vi "Aero_Tunnel_Monitor.vi"() -> ()   [LabVIEW 2012]
uses:
  ATE_Road_Data.ctl
  ATE_Machine_Status.ctl
  ATE_Road_Control.ctl
  ATE_Balance_Data.ctl
  ATE_Fan_Control.ctl
  ATE_Fan_Data.ctl
  Controls/Post_Process.ctl
  <vilib>/Platform/TimedLoop/XDataNode/timing_clust.ctl
  <vilib>/Platform/TimedLoop/XDataNode/nitl_modes.ctl
  <vilib>/Platform/TimedLoop/XDataNode/wakeup.ctl
  ADAM Client/Sub VIs/ADAM Controls/Update_scan_value.ctl
  Globals/Meas_global.vi
  <vilib>/Platform/TimedLoop/XDataNode/XDataNode.xnode
  <vilib>/Platform/TimedLoop/XDataNode/XDNodeRunTimeDep.lvlib
panel:
  out "Dem Tunnel Speed":dbl
  out "Paths":path[](array[path])
  out "error out":errorcluster
  out "Road Data REF":refnum<k21>="ni.var.psp://192.168.8.2/ATE_Shared_Variables/Road_Data"
  out "Road Control REF":refnum<k21>="ni.var.psp://192.168.8.2/ATE_Shared_Variables/Road_Control"
  out "Fan Data REF":refnum<k21>="ni.var.psp://192.168.8.2/ATE_Shared_Variables/Fan_Data"
  out "Fan Control REF":refnum<k21>="ni.var.psp://192.168.8.2/ATE_Shared_Variables/Fan_Control"
  out "Balance Data REF":refnum<k21>="ni.var.psp://192.168.8.2/ATE_Shared_Variables/Balance_Data"
  out "ATE_Machine Status REF":refnum<k21>="ni.var.psp://192.168.8.2/ATE_Shared_Variables/ATE_Machine_Status"
  in  "Stop Button":bool
  out "SMAD Temp":dbl=22.85
  out "First Loop? 3":bool
  out "First Loop? 2":bool
  out "First Loop?":bool=TRUE
  out "Fan Data":T1={"Fan Speed Dial (RPM)"=1.0, "Wind Speed Dial (m/s)"=0.0, "Wind Speed (m/s)"=0.0, "Fan Speed (RPM)"=1.0} {"Wind Speed Dial (m/s)" scale=0.0..45.0; "Fan Speed Dial (RPM)" scale=0.0..1000.0}
  out "Fan Control":T2={"Reset Pitot?"=FALSE, "Set Fan State"=FALSE, "Set Pressure"=1006.6041, "Set Fan Speed"=0.0, "Set Wind Speed Ratio"=0.0, "Tweak Change?"=FALSE, "Speed Change?"=FALSE}
  out "Balance_Data":T3={"%Lift"=28.01, "Lift"=185.018, "%Pitch"=22.34, "Pitch"=18.53, "%Drag"=2.21, "Drag"=4.327, "%Side"=-0.01, "Side"=-0.05, "%Yaw"=-2.47, "Yaw"=-0.307, "%Roll"=0.55, "Roll"=0.455} {"%Roll" scale=-100.0..100.0; "Roll" format="%5.1f Nm"; "%Yaw" scale=-100.0..100.0; "Yaw" format="%5.1f Nm"; "%Side" scale=-100.0..100.0; "Side" format="%5.1f N"; "%Drag" scale=-100.0..100.0; "Drag" format="%5.1f N"; "%Pitch" scale=-100.0..100.0; "Pitch" format="%5.1f Nm"; "%Lift" scale=-100.0..100.0; "Lift" format="%5.1f N"}
  in  "Road Control":T4 {"BL Suction Fan 2" scale=0.0..100.0; "BL Suction Fan 1" scale=0.0..100.0}
  out "ATE_Machine_Status":T5={"Loop Status"=FALSE, "Loop Frequency"=321.8613369862449, "Poor Loops"=0.0, "Pulse"=TRUE} {"Poor Loops" format="%0.2f %"; "Loop Frequency" format="%0.2f Hz"}
  out "Motor Enable":bool=TRUE
  out "Fan Watchdog":bool
  in  "Display Graph?":bool
  out "Belt Slip Warning":bool
  out "Road Enabled":bool
  out "Working Section Temperature":dbl=23.0
  out "Dem Road Speed":dbl
  in  "Balance Safety Limits":T6(array[cluster])=[{"Max +ve Range"=80, "Min -ve Range"=80, "Axis"="Lift"}, {"Max +ve Range"=80, "Min -ve Range"=80, "Axis"="Pitch"}, {"Max +ve Range"=120, "Min -ve Range"=120, "Axis"="Drag"}, {"Max +ve Range"=80, "Min -ve Range"=80, "Axis"="Side"}, {"Max +ve Range"=120, "Min -ve Range"=120, "Axis"="Yaw"}, {"Max +ve Range"=80, "Min -ve Range"=80, "Axis"="Roll"}]
  in  "Menu Ring":u16(ring) items=["Lift", "Pitch", "Drag", "Side", "Yaw", "Roll"]
  out "Waveform Chart":dbl(graph)
  out "OGI Client Loop Status":T5={"Loop Status"=FALSE, "Loop Frequency"=341.33991618739697, "Poor Loops"=1.2012012012012012, "Pulse"=FALSE} {"Poor Loops" format="%0.2f %"; "Loop Frequency" format="%0.2f Hz"}
  out "Road_Data":T7 {"Road Speed" scale=0.0..50.0; "Yaw Angle" scale=-5.0..5.0}
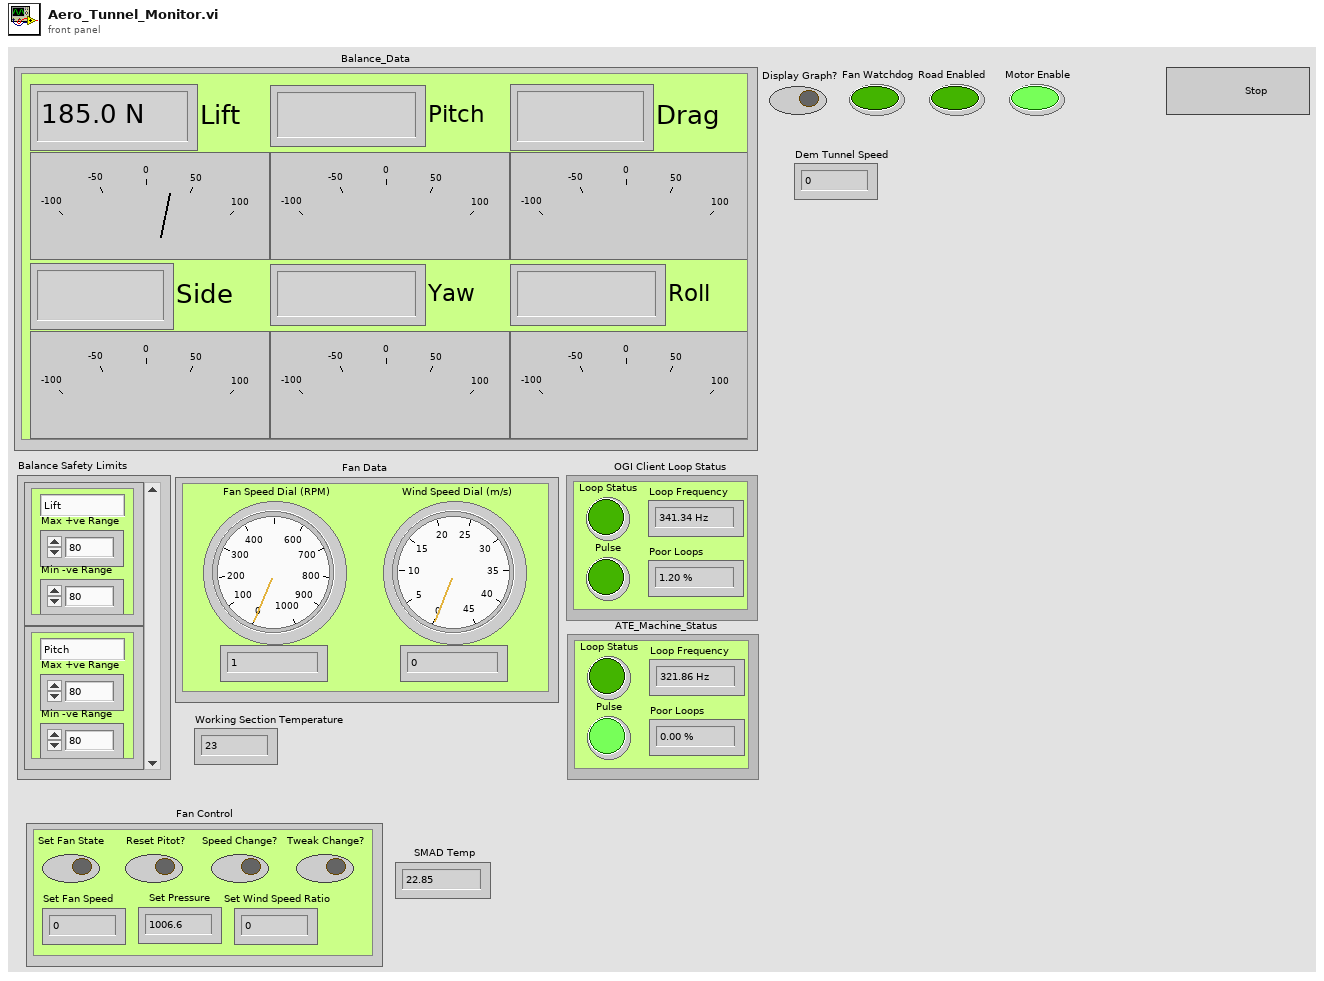
[diagram p1: front panel]
types:
  T1 = cluster{"Fan Speed Dial (RPM)":dbl, "Wind Speed Dial (m/s)":dbl, "Wind Speed (m/s)":dbl, "Fan Speed (RPM)":dbl}
  T2 = typedef "ATE_Fan_Control.ctl" = cluster{"Reset Pitot?":bool, "Set Fan State":bool, "Set Pressure":dbl, "Set Fan Speed":dbl, "Set Wind Speed Ratio":dbl, "Tweak Change?":bool, "Speed Change?":bool}
  T3 = typedef "ATE_Balance_Data.ctl" = cluster{"%Lift":dbl, "Lift":dbl, "%Pitch":dbl, "Pitch":dbl, "%Drag":dbl, "Drag":dbl, "%Side":dbl, "Side":dbl, "%Yaw":dbl, "Yaw":dbl, "%Roll":dbl, "Roll":dbl}
  T4 = typedef "ATE_Road_Control.ctl" = cluster{"Sync to Wind":bool, "Start Drive":bool, "Stop Drive":bool, "BL Suction Fan 1":i32, "BL Suction Fan 2":i32, "Set Yaw Angle":dbl, "Road Active?":bool}
  T5 = typedef "ATE_Machine_Status.ctl" = cluster{"Loop Status":bool, "Loop Frequency":dbl, "Poor Loops":dbl, "Pulse":bool}
  T6 = cluster{"Max +ve Range":i32, "Min -ve Range":i32, "Axis":string}[]
  T7 = typedef "ATE_Road_Data.ctl" = cluster{"Road Information":string, "Road Status":string, "Yaw Angle":dbl, "Road Speed":dbl}
  T8 = typedef "Post_Process.ctl" = enum16{"Take New Data", "Post Process Raw Data File"}
  T9 = typedef "Update_scan_value.ctl" = cluster{"Channel Name":string, "New Value":dbl}
  T10 = typedef "XDNodeRunTimeDep.lvlib/timing_clust.ctl" = cluster{"Expected End [f-1]":u64, "Actual End [f-1]":u64, "Finished Late? [f-1]":bool, "Expected End [i-1]":u64, "Actual End [i-1]":u64, "Finished Late? [i-1]":bool, "Expected Start [i]":u64, "Actual Start [i]":u64, "Expected Start [f]":u64, "Actual Start [f]":u64, "Source Name":string, "Structure Name":string, "Period":i64, "Deadline":i64, "Offset":i64, "Start":i64, "Priority":i32, "Timeout":i32, "Mode":T11, "Wakeup Reason":T12, "Error":errorcluster, "Source Type":string, "Secondary Source Type":string, "Global End Time":u64, "Global Start Time":u64, "Frame Duration":u64, "Iteration Duration":u64, "Assigned CPU":i32, "I/O Scan Engine Mode":u32}
  T11 = typedef "XDNodeRunTimeDep.lvlib/nitl_modes.ctl" = enum32{"No Change", "Process missed periods, maintain original phase", "Discard missed periods, maintain original phase", "Process missed periods, ignore original phase", "Discard missed periods, ignore original phase"}
  T12 = typedef "XDNodeRunTimeDep.lvlib/wakeup.ctl" = enum32{"Normal", "Aborted", "Asynchronous wakeup", "Timing source error", "Timed loop error", "Timeout"}
  T13 = typedef "ATE_Fan_Data.ctl" = cluster{"Fan Speed (RPM)":dbl, "Wind Speed (m/s)":dbl, "SMAD Data":string}
  T14 = typedef "LVDateTimeRec.ctl" = cluster{"fractional second":dbl, "second":i32, "minute":i32, "hour":i32, "day of month":i32, "month":i32, "year":i32, "day of week":i32, "day of year":i32, "DST":i32}
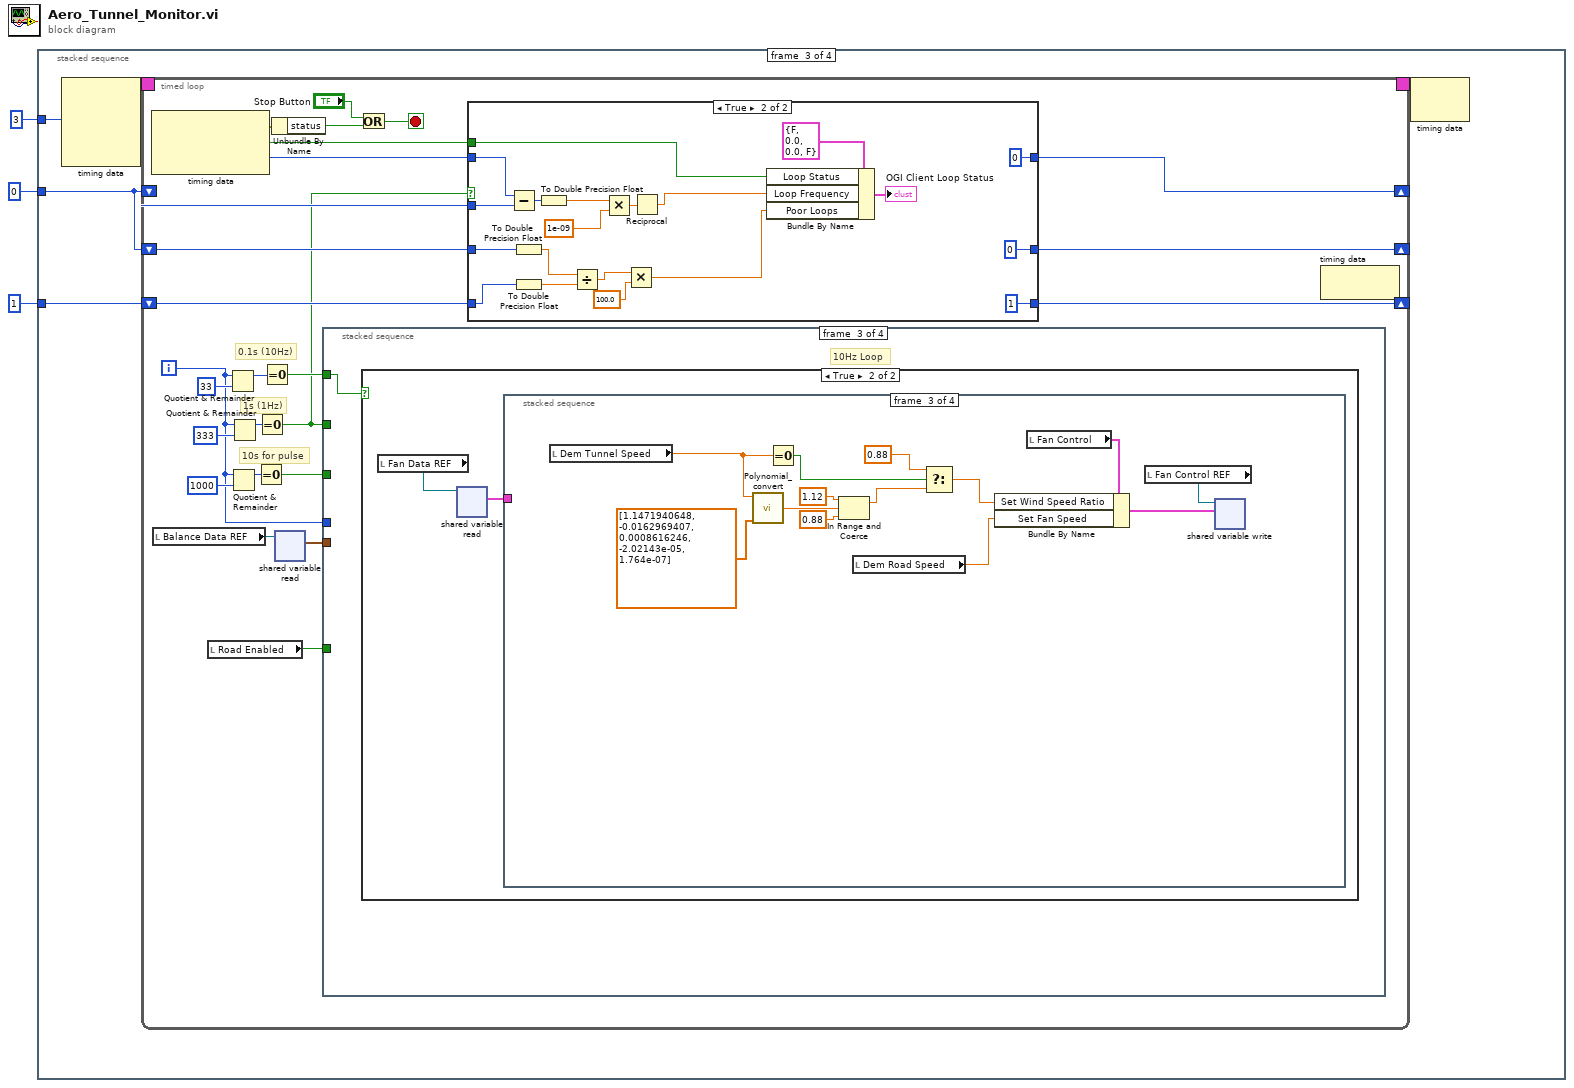
[diagram p0: block diagram]
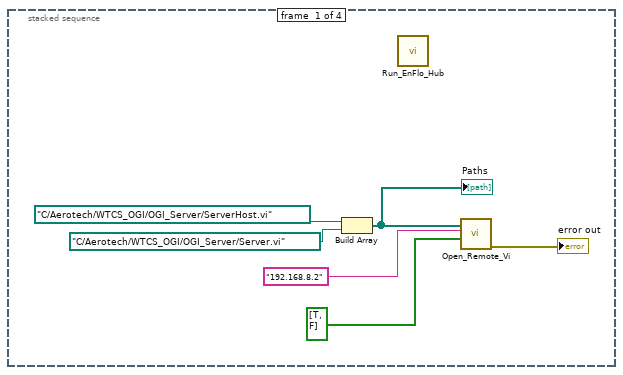
[diagram p2: hidden frame]
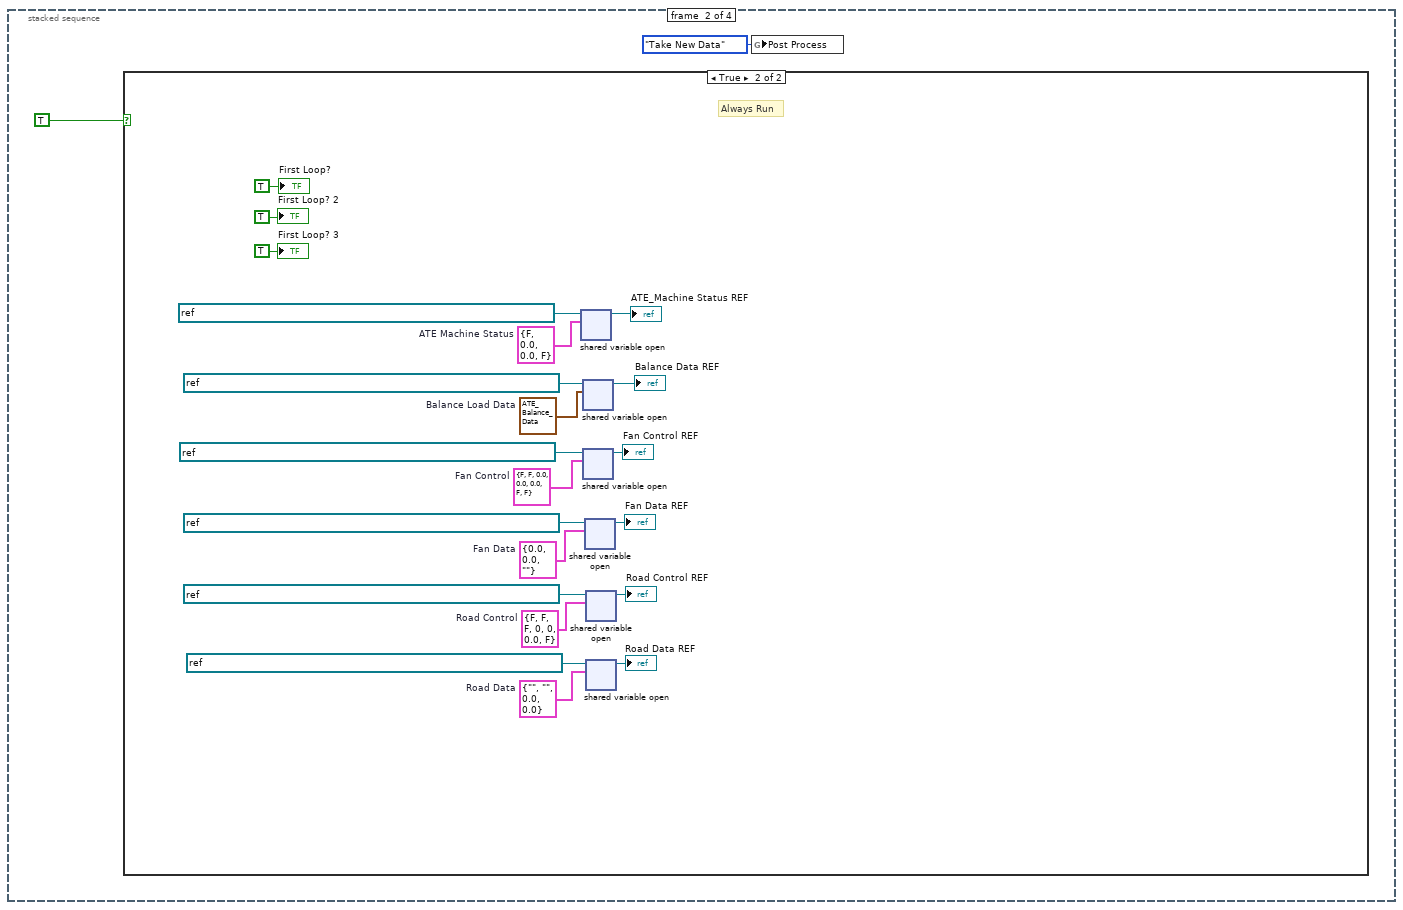
[diagram p3: hidden frame]
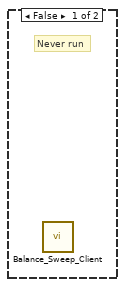
[diagram p4: hidden frame]
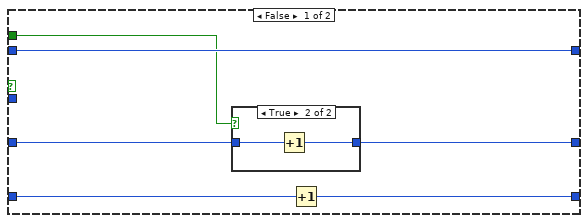
[diagram p5: hidden frame]
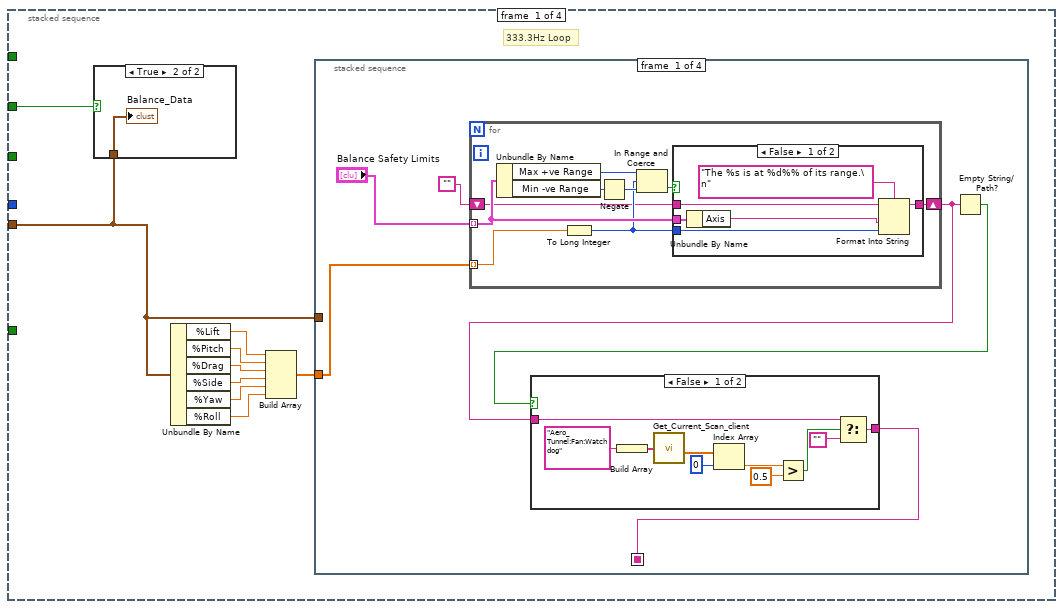
[diagram p7: hidden frame]
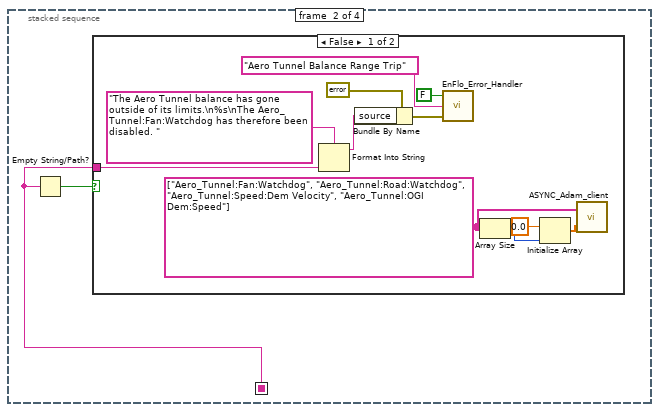
[diagram p11: hidden frame]
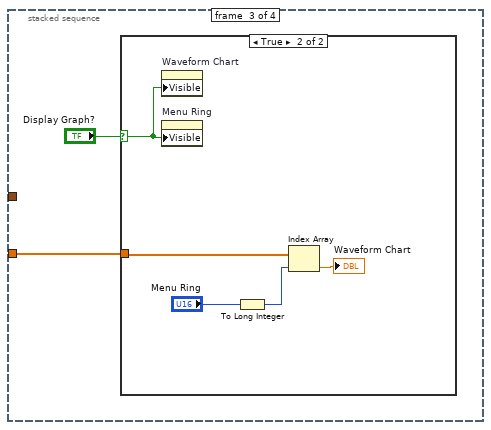
[diagram p13: hidden frame]
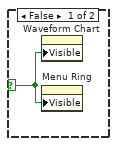
[diagram p14: hidden frame]
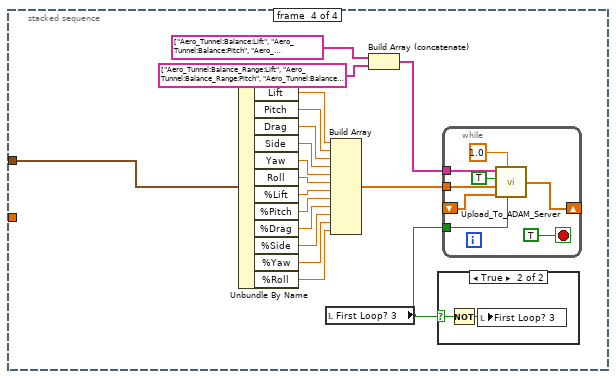
[diagram p15: hidden frame]
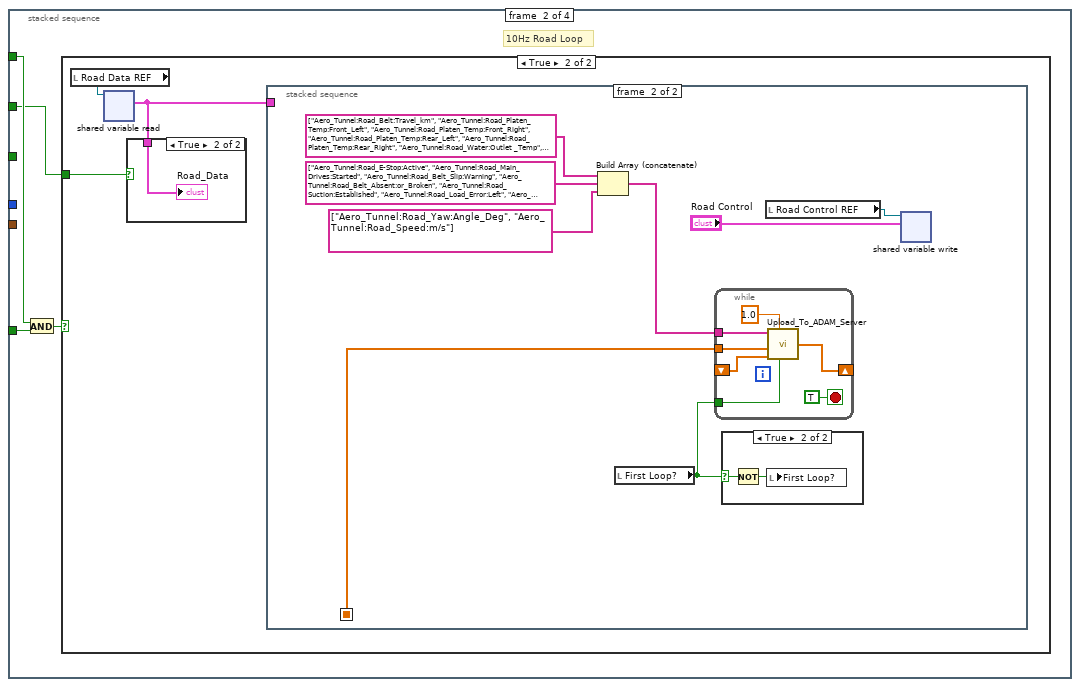
[diagram p17: hidden frame]
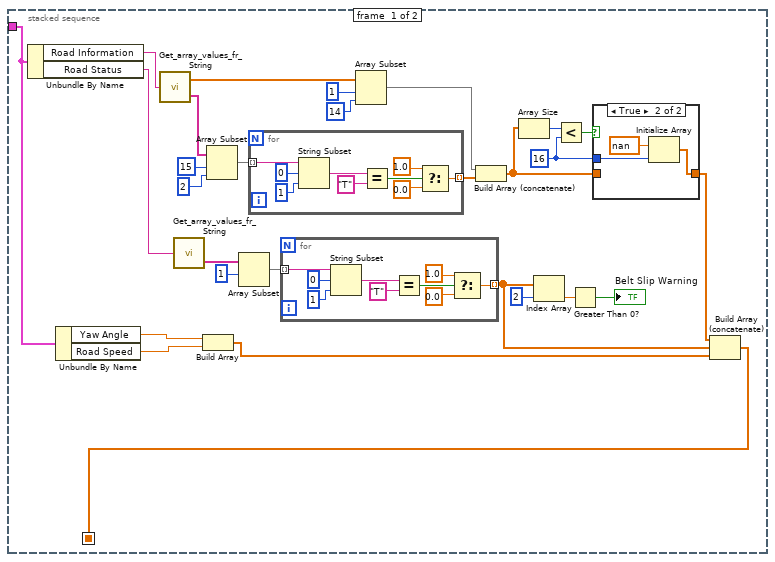
[diagram p20: hidden frame]
diagram:
  n1 = stacked-sequence {
    tunnel: i64 3 ("Period") -> [_ _ w35 _]
    tunnel: i64 0 ("Period") -> [_ _ w34 _]
    tunnel: i64 1 ("Period") -> [_ _ w33 _]
    frame #0 {
      n2 = Build Array(path "C:/Aerotech/WTCS_OGI/OGI_Server/ServerHost.vi" ("VI Path"), path "C:/Aerotech/WTCS_OGI/OGI_Server/Server.vi" ("VI Path")) -> (w6:path[])
      "Paths" <- w6
      n3 = call "Run_EnFlo_Hub.vi"() -> ()  [unwired: 8 in]
      n4 = call "Open_Remote_Vi.vi"("Run Minimised?"=bool[] [TRUE, FALSE], "Remote IP"="192.168.8.2", "Vi Path"=w6) -> ("error out"=→"error out":errorcluster)  [unwired: 8 in]
    }
    frame #1 {
      n5 = case shown="True" TRUE {
        frame False {
          # "Never run"
          n6 = call "Balance_Sweep_Client.vi"() -> ()  [unwired: 5 in, 1 out]
        }
        frame True {
          w16 = T7 {"Road Information"="", "Road Status"="", "Yaw Angle"=0.0, "Road Speed"=0.0}  # Road Data
          w18 = T4 {"Sync to Wind"=FALSE, "Start Drive"=FALSE, "Stop Drive"=FALSE, "BL Suction Fan 1"=0, "BL Suction Fan 2"=0, "Set Yaw Angle"=0.0, "Road Active?"=FALSE}  # Road Control
          w28 = T5 {"Loop Status"=FALSE, "Loop Frequency"=0.0, "Poor Loops"=0.0, "Pulse"=FALSE}  # ATE Machine Status
          w20 = T13 {"Fan Speed (RPM)"=0.0, "Wind Speed (m/s)"=0.0, "SMAD Data"=""}  # Fan Data
          w22 = T2 {"Reset Pitot?"=FALSE, "Set Fan State"=FALSE, "Set Pressure"=0.0, "Set Fan Speed"=0.0, "Set Wind Speed Ratio"=0.0, "Tweak Change?"=FALSE, "Speed Change?"=FALSE}  # Fan Control
          w26 = T3 {"%Lift"=0.0, "Lift"=0.0, "%Pitch"=0.0, "Pitch"=0.0, "%Drag"=0.0, "Drag"=0.0, "%Side"=0.0, "Side"=0.0, "%Yaw"=0.0, "Yaw"=0.0, "%Roll"=0.0, "Roll"=0.0}  # Balance Load Data
          # "Always Run"
          n7 = shared-variable-open(refnum<k21> "ni.var.psp://192.168.8.2/ATE_Shared_Variables/ATE_Machine_Status" ("shared variable refnum in"), w28) -> (→"ATE_Machine Status REF":refnum<k21>)  [unwired: 2 in, 1 out]
          n8 = shared-variable-open(refnum<k21> "ni.var.psp://192.168.8.2/ATE_Shared_Variables/Balance_Data" ("shared variable refnum in"), w26) -> (→"Balance Data REF":refnum<k21>)  [unwired: 2 in, 1 out]
          n9 = shared-variable-open(refnum<k21> "ni.var.psp://192.168.8.2/ATE_Shared_Variables/Fan_Control" ("shared variable refnum in"), w22) -> (→"Fan Control REF":refnum<k21>)  [unwired: 2 in, 1 out]
          n10 = shared-variable-open(refnum<k21> "ni.var.psp://192.168.8.2/ATE_Shared_Variables/Fan_Data" ("shared variable refnum in"), w20) -> (→"Fan Data REF":refnum<k21>)  [unwired: 2 in, 1 out]
          n11 = shared-variable-open(refnum<k21> "ni.var.psp://192.168.8.2/ATE_Shared_Variables/Road_Control" ("shared variable refnum in"), w18) -> (→"Road Control REF":refnum<k21>)  [unwired: 2 in, 1 out]
          n12 = shared-variable-open(refnum<k21> "ni.var.psp://192.168.8.2/ATE_Shared_Variables/Road_Data" ("shared variable refnum in"), w16) -> (→"Road Data REF":refnum<k21>)  [unwired: 2 in, 1 out]
          "First Loop?" <- TRUE
          "First Loop? 2" <- TRUE
          "First Loop? 3" <- TRUE
        }
      }
      n13 = global write "Meas_global.vi" "Post Process"(Post_Process."Take New Data" ("Post Process")) -> ()
    }
    frame #2 {
      n14 = node-c288(w35) -> (w37:T10)  [unwired: 3 in]
      n15 = timed-loop {
        timing: w37 -> [_]
        timing-out: [_] -> w36
        shift-right: [w44] -> _
        shift-left: w34 -> [w51]
        shift-right: [w46] -> _
        shift-left: w34 -> [w58]
        shift-right: [w49] -> _
        shift-left: w33 -> [w48]
        i -> [w38]
        stop <- w41 stop-if-true
        # "10s for pulse"
        # "1s (1Hz)"
        # "0.1s (10Hz)"
        n16 = node-c288() -> (w62:errorcluster, w47:bool, w59:i64)  [unwired: 1 in]
        n17 = local read "Balance Data REF"() -> (w40:refnum<k21>)
        n18 = local read "Road Enabled"() -> (w55:bool)
        n19 = Quotient & Remainder(x=w38, y=33) -> (x-y*floor(x/y)=w60:i32)  [unwired: 1 out]
        n20 = Quotient & Remainder(x=w38, y=1000) -> (x-y*floor(x/y)=w56:i32)  [unwired: 1 out]
        n21 = Quotient & Remainder(x=w38, y=333) -> (x-y*floor(x/y)=w61:i32)  [unwired: 1 out]
        n22 = Equal To 0?(x=w56) -> (x = 0?=w50:bool)
        n23 = Equal To 0?(x=w61) -> (x = 0?=w45:bool)
        n24 = Equal To 0?(x=w60) -> (x = 0?=w57:bool)
        n25 = Unbundle By Name(w62) -> ("status"=w43:bool)
        n26 = shared-variable-read(w40) -> (w39:T3)  [unwired: 1 in, 3 out]
        n27 = stacked-sequence {
          tunnel: w57 -> [_ w185 w259 _]
          tunnel: w45 -> [w93 w184 _ _]
          tunnel: w55 -> [_ w186 _ _]
          tunnel: w50 -> [_ _ _ w360]
          tunnel: w39 -> [w92 _ _ _]
          tunnel: w38 -> [_ _ _ w359]
          frame #0 {
            # "333.3Hz Loop"
            n28 = case shown="True" w93 {
              tunnel: w92 -> [_ w101]
              frame False {
              }
              frame True {
                "Balance_Data" <- w101
              }
            }
            n29 = Unbundle By Name(w92) -> ("%Lift"=w99:dbl, "%Pitch"=w98:dbl, "%Drag"=w97:dbl, "%Side"=w96:dbl, "%Yaw"=w95:dbl, "%Roll"=w94:dbl)
            n30 = Build Array(w99, w98, w97, w96, w95, w94) -> (w100:dbl[])
            n31 = stacked-sequence {
              seq-local: [w102 _ _ _] -> [_ w135 _ _]
              tunnel: w100 -> [w106 _ w148 _]
              tunnel: w92 -> [_ _ _ w159]
              frame #0 {
                n32 = for {
                  tunnel: "Balance Safety Limits" -> [w122] mode=indexing
                  tunnel: w106 -> [w125] mode=indexing
                  shift-right: [w119] -> w104
                  shift-left: "" -> [w120]
                  n33 = Unbundle By Name(w122) -> ("Max +ve Range"=w127:i32, "Min -ve Range"=w126:i32)
                  n34 = To Long Integer(number=w125) -> (32bit integer=w121:i32)
                  n35 = Negate(x=w126) -> (-x=w124:i32)
                  n36 = In Range and Coerce(upper limit=w127, x=w121, lower limit=w124) -> (In Range?=w123:bool)  [unwired: 1 out]
                  n37 = case shown="False" w123 {
                    tunnel: w122 -> [w133 _]
                    tunnel: w121 -> [w131 _]
                    tunnel: w120 -> [w129 w134]
                    tunnel: [w128 w134] -> w119
                    frame False {
                      n38 = Unbundle By Name(w133) -> ("Axis"=w132:string)
                      n39 = Format Into String(format string="The %s is at %d%% of its range.\n", initial string=w129, w132, w131) -> (resulting string=w128:string)  [unwired: 1 in, 1 out]
                    }
                    frame True {
                    }
                  }
                }
                n40 = Empty String/Path?(string/path=w104) -> (empty?=w105:bool)
                n41 = case shown="False" w105 {
                  tunnel: w104 -> [w110 w118]
                  tunnel: [w108 w118] -> w102
                  frame False {
                    n42 = Build Array("Aero_Tunnel:Fan:Watchdog") -> (w117:string[])
                    n43 = call "Get_Current_Scan_client.vi"("ADAM Ch Names"=w117) -> ("Numerical Values"=w115:dbl[])  [unwired: 1 in, 2 out]
                    n44 = Index Array(array=w115, index=0) -> (element=w113:dbl)
                    n45 = Greater?(x=w113, y=0.5) -> (0:w111:bool)
                    n46 = Select(t=w110, s=w111, f="") -> (s? t:f=w108:string)
                  }
                  frame True {
                  }
                }
              }
              frame #1 {
                n47 = Empty String/Path?(string/path=w135) -> (empty?=w136:bool)
                n48 = case shown="False" w136 {
                  tunnel: w135 -> [w141 _]
                  frame False {
                    w140 = string[] ["Aero_Tunnel:Fan:Watchdog", "Aero_Tunnel:Road:Watchdog", "Aero_Tunnel:Speed:Dem Velocity", "Aero_Tunnel:OGI Dem:Speed"] ("Channel Names")
                    n49 = Format Into String(format string="The Aero Tunnel balance has gone outside of its limits.\n%s\nThe Aero_Tunnel:Fan:Watchdog has therefore been disabled. ", w141) -> (resulting string=w142:string)  [unwired: 2 in, 1 out]
                    n50 = Bundle By Name(cluster=errorcluster {"status"=TRUE, "code"=0, "source"=""} ("error in (no error)"), "source"=w142) -> (w144:errorcluster)
                    n51 = call "EnFlo_Error_Handler.vi"("error in (no error)"=w144, "Error Type"="Aero Tunnel Balance Range Trip", "Dialog Box (T)"=FALSE) -> ()  [unwired: 3 out]
                    n52 = Array Size(array=w140) -> (size(s)=w139:i32)
                    n53 = Initialize Array(0.0, w139) -> (w137:dbl[])
                    n54 = call "ASYNC_Adam_client.vi"("Values"=w137, "Channel Names"=w140) -> ()  [unwired: 2 out]
                  }
                  frame True {
                  }
                }
              }
              frame #2 {
                n55 = case shown="True" "Display Graph?" {
                  selector: "Display Graph?" -> [w150 w153]
                  tunnel: w148 -> [_ w151]
                  frame False {
                    n56 = property on="Waveform Chart" class="WFChart (strict)"("Visible"=w150) -> ()  [unwired: 2 in, 2 out]
                    n57 = property on="Menu Ring" class="Ring (strict)"("Visible"=w150) -> ()  [unwired: 2 in, 2 out]
                  }
                  frame True {
                    n58 = property on="Waveform Chart" class="WFChart (strict)"("Visible"=w153) -> ()  [unwired: 2 in, 2 out]
                    n59 = property on="Menu Ring" class="Ring (strict)"("Visible"=w153) -> ()  [unwired: 2 in, 2 out]
                    n60 = To Long Integer(number="Menu Ring") -> (32bit integer=w152:i32)
                    n61 = Index Array(array=w151, index=w152) -> (element=→"Waveform Chart":dbl)
                  }
                }
              }
              frame #3 {
                n62 = Unbundle By Name(w159) -> ("Lift"=w173:dbl, "Pitch"=w172:dbl, "Drag"=w171:dbl, "Side"=w170:dbl, "Yaw"=w169:dbl, "Roll"=w168:dbl, "%Lift"=w167:dbl, "%Pitch"=w166:dbl, "%Drag"=w165:dbl, "%Side"=w164:dbl, "%Yaw"=w163:dbl, "%Roll"=w162:dbl)
                n63 = local read "First Loop? 3"() -> (w156:bool)
                n64 = Build Array(w173, w172, w171, w170, w169, w168, w167, w166, w165, w164, w163, w162) -> (w157:dbl[])
                n65 = Build Array (concatenate)(string[] ["Aero_Tunnel:Balance:Lift", "Aero_Tunnel:Balance:Pitch", "Aero_Tunnel:Balance:Drag", "Aero_Tunnel:Balance:Side-Force", "Aero_Tunnel:Balance:Yaw", "Aero_Tunnel:Balance:Roll"] ("Channel Names"), string[] ["Aero_Tunnel:Balance_Range:Lift", "Aero_Tunnel:Balance_Range:Pitch", "Aero_Tunnel:Balance_Range:Drag", "Aero_Tunnel:Balance_Range:Side-Force", "Aero_Tunnel:Balance_Range:Yaw", "Aero_Tunnel:Balance_Range:Roll"] ("Channel Names")) -> (w158:string[])
                n66 = case shown="True" w156 {
                  selector: w156 -> [_ w175]
                  frame False {
                  }
                  frame True {
                    n67 = Not(x=w175) -> (.not. x?=w174:bool)
                    n68 = local write "First Loop? 3"(w174) -> ()
                  }
                }
                n69 = while {
                  tunnel: w158 -> [w183]
                  tunnel: w157 -> [w181]
                  shift-right: [w179] -> _
                  shift-left: _ -> [w178]
                  tunnel: w156 -> [w177]
                  stop <- TRUE stop-if-true
                  n70 = call "Upload_To_ADAM_Server.vi"("First Loop"=w177, "Averaging Period (s)"=1.0, "Shift In"=w178, "Channel Values"=w181, "Give Variance"=TRUE, "Channel Names"=w183) -> ("Shift Out"=w179:dbl[])
                }
              }
            }
          }
          frame #1 {
            # "10Hz Road Loop"
            n71 = And(x=w185, y=w186) -> (x .and. y?=w187:bool)
            n72 = case shown="True" w187 {
              tunnel: w184 -> [_ w190]
              frame False {
                # "Do Nothing"
              }
              frame True {
                n73 = local read "Road Data REF"() -> (w189:refnum<k21>)
                n74 = shared-variable-read(w189) -> (w188:T7)  [unwired: 1 in, 3 out]
                n75 = case shown="True" w190 {
                  tunnel: w188 -> [_ w191]
                  frame False {
                  }
                  frame True {
                    "Road_Data" <- w191
                  }
                }
                n76 = stacked-sequence {
                  seq-local: [w196 _] -> [_ w245]
                  tunnel: w188 -> [w195 _]
                  frame #0 {
                    w217 = 16 ("y")
                    n77 = Unbundle By Name(w195) -> ("Road Information"=w206:string, "Road Status"=w200:string)
                    n78 = Unbundle By Name(w195) -> ("Yaw Angle"=w194:dbl, "Road Speed"=w193:dbl)
                    n79 = call "Get_array_values_fr_String.vi"("String Value"=w206) -> ("Numeric Array"=w218:dbl[], "String array"=w214:string[])
                    n80 = call "Get_array_values_fr_String.vi"("String Value"=w200) -> ("String array"=w203:string[])  [unwired: 1 out]
                    n81 = Build Array(w194, w193) -> (w192:dbl[])
                    n82 = Array Subset(array=w214, index=15, length=2) -> (w211:string[])
                    n83 = Array Subset(array=w203, index=1) -> (w205:string[])  [unwired: 1 in]
                    n84 = for {
                      tunnel: w211 -> [w239] mode=indexing
                      tunnel: [w233] -> w212 mode=indexing
                      n85 = String Subset(string=w239, offset (0)=0, length (rest)=1 ("length (rest)")) -> (substring=w238:string)
                      n86 = Equal?(x=w238, y="T") -> (x = y?=w236:bool)
                      n87 = Select(t=1.0, s=w236, f=0.0) -> (s? t:f=w233:dbl)
                    }
                    n88 = for {
                      tunnel: [w221] -> w197 mode=indexing
                      tunnel: w205 -> [w220] mode=indexing
                      n89 = String Subset(string=w220, offset (0)=0, length (rest)=1 ("length (rest)")) -> (substring=w226:string)
                      n90 = Equal?(x=w226, y="T") -> (x = y?=w224:bool)
                      n91 = Select(t=1.0, s=w224, f=0.0) -> (s? t:f=w221:dbl)
                    }
                    n92 = Array Subset(array=w218, index=1, length=14) -> (w213:dbl[])
                    n93 = Build Array (concatenate)(w213, w212) -> (w219:dbl[])
                    n94 = Array Size(array=w219) -> (size(s)=w215:i32)
                    n95 = Index Array(array=w197, index=2) -> (element=w202:dbl)
                    n96 = Less?(x=w215, y=w217) -> (x < y?=w216:bool)
                    n97 = Greater Than 0?(x=w202) -> (x > 0?=→"Belt Slip Warning":bool)
                    n98 = case shown="True" w216 {
                      tunnel: [w229 w232] -> w198
                      tunnel: w219 -> [w229 _]
                      tunnel: w217 -> [_ w230]
                      frame False {
                      }
                      frame True {
                        n99 = Initialize Array(nan, w230) -> (w232:dbl[])
                      }
                    }
                    n100 = Build Array (concatenate)(w198, w197, w192) -> (w196:dbl[])
                  }
                  frame #1 {
                    n101 = Build Array (concatenate)(string[] ["Aero_Tunnel:Road_Belt:Travel_km", "Aero_Tunnel:Road_Platen_Temp:Front_Left", "Aero_Tunnel:Road_Platen_Temp:Front_Right", "Aero_Tunnel:Road_Platen_Temp:Rear_Left", "Aero_Tunnel:Road_Platen_Temp:Rear_Right", "Aero_Tunnel:Road_Water:Outlet _Temp", "Aero_Tunnel:Road_Water:Inlet _Temp", "Aero_Tunnel:Road_Suction:Front", "Aero_Tunnel:Road_Suction:Middle", "Aero_Tunnel:Road_Suction:Rear", "Aero_Tunnel:Road_BL_Suction:Primary", "Aero_Tunnel:Road_BL_Suction:Secondary", "Aero_Tunnel:Road_LoadCell:Left", "Aero_Tunnel:Road_LoadCell:Right", "Aero_Tunnel:Road_Water_High:Temp_Alarm", "Aero_Tunnel:Road_Platen_High:Temp_Alarm"] ("Channel Names"), string[] ["Aero_Tunnel:Road_E-Stop:Active", "Aero_Tunnel:Road_Main_Drives:Started", "Aero_Tunnel:Road_Belt_Slip:Warning", "Aero_Tunnel:Road_Belt_Absent:or_Broken", "Aero_Tunnel:Road_Suction:Established", "Aero_Tunnel:Road_Load_Error:Left", "Aero_Tunnel:Road_Load_Error:Right", "Aero_Tunnel:Road_Water_Alarm:Active", "Aero_Tunnel:Road_Platen_Alarm:Active"] ("Channel Names"), string[] ["Aero_Tunnel:Road_Yaw:Angle_Deg", "Aero_Tunnel:Road_Speed:m/s"] ("Channel Names")) -> (w246:string[])
                    n102 = local read "First Loop?"() -> (w244:bool)
                    n103 = while {
                      tunnel: w246 -> [w258]
                      tunnel: w245 -> [w256]
                      shift-right: [w254] -> _
                      shift-left: _ -> [w253]
                      tunnel: w244 -> [w252]
                      stop <- TRUE stop-if-true
                      n104 = call "Upload_To_ADAM_Server.vi"("First Loop"=w252, "Averaging Period (s)"=1.0, "Shift In"=w253, "Channel Values"=w256, "Channel Names"=w258) -> ("Shift Out"=w254:dbl[])  [unwired: 1 in]
                    }
                    n105 = case shown="True" w244 {
                      selector: w244 -> [_ w251]
                      frame False {
                      }
                      frame True {
                        n106 = Not(x=w251) -> (.not. x?=w250:bool)
                        n107 = local write "First Loop?"(w250) -> ()
                      }
                    }
                    n108 = local read "Road Control REF"() -> (w243:refnum<k21>)
                    n109 = shared-variable-write(w243, "Road Control") -> ()  [unwired: 1 in, 2 out]
                  }
                }
              }
            }
          }
          frame #2 {
            # "10Hz Loop"
            n110 = case shown="True" w259 {
              frame False {
                # "Do Nothing"
              }
              frame True {
                n111 = local read "Fan Data REF"() -> (w261:refnum<k21>)
                n112 = shared-variable-read(w261) -> (w260:T13)  [unwired: 1 in, 3 out]
                n113 = stacked-sequence {
                  tunnel: w260 -> [w284 _ _ _]
                  frame #0 {
                    w270 = 17 ("y")
                    n114 = Unbundle By Name(w284) -> ("Wind Speed (m/s)"=w266:dbl, "Fan Speed (RPM)"=w267:dbl, "SMAD Data"=w268:string)
                    n115 = call "Get_array_values_fr_String.vi"("String Value"=w268) -> ("Numeric Array"=w271:dbl[], "String array"=w274:string[])
                    n116 = Array Size(array=w274) -> (size(s)=w275:i32)
                    n117 = Less?(x=w275, y=w270) -> (x < y?=w273:bool)
                    n118 = case shown="True" w273 {
                      tunnel: [w289 w292] -> w272
                      tunnel: w271 -> [w289 _]
                      tunnel: w270 -> [_ w290]
                      frame False {
                      }
                      frame True {
                        n119 = Initialize Array(nan, w290) -> (w292:dbl[])
                      }
                    }
                    n120 = Bundle By Name(cluster=T1 {"Fan Speed Dial (RPM)"=143.0, "Wind Speed Dial (m/s)"=4.76, "Wind Speed (m/s)"=0.0, "Fan Speed (RPM)"=0.0} ("Fan Data"), "Wind Speed Dial (m/s)"=w266, "Fan Speed Dial (RPM)"=w267, "Wind Speed (m/s)"=w266, "Fan Speed (RPM)"=w267) -> (→"Fan Data":T1)
                    n121 = Index Array(array=w272, index=16) -> (element=w262:dbl)
                    "SMAD Temp" <- w262
                    n122 = Index Array(array=w272, index=1) -> (element=w281:dbl)
                    n123 = Index Array(array=w272, index=11) -> (element=w279:dbl)
                    n124 = Less?(x=w279, y=100.0) -> (x < y?=w277:bool)
                    n125 = Boolean To (0,1)(Boolean=w277) -> (0, 1=w276:i16)
                    n126 = Build Array(w262, w281, w276) -> (w269:dbl[])
                    n127 = local read "First Loop? 2"() -> (w265:bool)
                    n128 = Build Array (concatenate)(w266, w267, w269) -> (w285:dbl[])
                    n129 = case shown="True" w265 {
                      selector: w265 -> [_ w288]
                      frame False {
                      }
                      frame True {
                        n130 = Not(x=w288) -> (.not. x?=w287:bool)
                        n131 = local write "First Loop? 2"(w287) -> ()
                      }
                    }
                    n132 = while {
                      tunnel: string[] ["Aero_Tunnel:Speed:Meas Velocity", "Aero_Tunnel:Fan:RPM", "Aero_Tunnel:SmAD:Temp", "Aero_Tunnel:Pitot tube:Voltage", "Aero_Tunnel:Drive:Ready"] ("Channel Names") -> [w299]
                      tunnel: w285 -> [w297]
                      shift-right: [w296] -> _
                      shift-left: _ -> [w295]
                      tunnel: w265 -> [w293]
                      stop <- TRUE stop-if-true
                      n133 = call "Upload_To_ADAM_Server.vi"("First Loop"=w293, "Averaging Period (s)"=1.0, "Shift In"=w295, "Channel Values"=w297, "Channel Names"=w299) -> ("Shift Out"=w296:dbl[])  [unwired: 1 in]
                    }
                  }
                  frame #1 {
                    n134 = call "Get_Current_Scan_client.vi"("ADAM Ch Names"=string[] ["Aero_Tunnel:Road:Dem_Velocity", "Froude:NPL:Atmos_Press", "Aero_Tunnel:Motor:Enable", "Aero_Tunnel:Thermistor:Temp", "Aero_Tunnel:Fan:Watchdog", "Aero_Tunnel:Rolling_Road:Enable", "Aero_Tunnel:Speed:Dem Velocity"] ("appended array")) -> ("Numerical Values"=w325:dbl[])  [unwired: 1 in, 2 out]
                    n135 = Index Array(array=w325) -> (element #1=w314:dbl, element #2=w318:dbl, element #3=w320:dbl, element #4=→"Working Section Temperature":dbl, element #5=w302:dbl, element #6=w301:dbl, element #7=→"Dem Tunnel Speed":dbl)  [unwired: 7 in]
                    "Dem Road Speed" <- w314
                    n136 = local read "Dem Road Speed"() -> (w317:dbl)
                    n137 = To Unsigned Word Integer(number=w302) -> (unsigned 16bit integer=w323:u16)
                    n138 = To Unsigned Word Integer(number=w301) -> (unsigned 16bit integer=w324:u16)
                    n139 = Greater?(x=w314, y=0.2) -> (0:w313:bool)
                    n140 = Not Equal To 0?(x=w324) -> (x != 0?=w310:bool)
                    "Road Enabled" <- w310
                    n141 = Not Equal To 0?(x=w323) -> (x != 0?=→"Fan Watchdog":bool)
                    n142 = Greater?(x=w320, y=0.5) -> (0:w312:bool)
                    "Motor Enable" <- w312
                    n143 = Not Equal?(x=w314, y=w317) -> (x != y?=w316:bool)
                    n144 = Not(x=w312) -> (.not. x?=w311:bool)
                    n145 = local read "Road Control"() -> (w305:T4)
                    n146 = Bundle By Name(cluster=w305, "Road Active?"=w310) -> (w309:T4)
                    n147 = Bundle By Name(cluster=T2 {"Reset Pitot?"=FALSE, "Set Fan State"=FALSE, "Set Pressure"=0.0, "Set Fan Speed"=0.0, "Set Wind Speed Ratio"=0.0, "Tweak Change?"=FALSE, "Speed Change?"=FALSE} ("Fan Control"), "Set Fan State"=w313, "Speed Change?"=w316, "Set Pressure"=w318, "Reset Pitot?"=w311, "Tweak Change?"=FALSE) -> (w306:T2)
                    "Fan Control" <- w306
                    n148 = local read "Road Control REF"() -> (w308:refnum<k21>)
                    n149 = local read "Fan Control REF"() -> (w307:refnum<k21>)
                    n150 = property on="Road_Data" class="Clust (strict)"("Visible"=w310) -> ()  [unwired: 2 in, 2 out]
                    n151 = property on="Road Control" class="Clust (strict)"("Visible"=w310) -> ()  [unwired: 2 in, 2 out]
                    n152 = property on="Belt Slip Warning" class="Bool (strict)"("Visible"=w310) -> ()  [unwired: 2 in, 2 out]
                    n153 = shared-variable-write(w307, w306) -> ()  [unwired: 1 in, 2 out]
                    n154 = shared-variable-write(w308, w309) -> ()  [unwired: 1 in, 2 out]
                  }
                  frame #2 {
                    n155 = local read "Dem Tunnel Speed"() -> (w332:dbl)
                    n156 = call "Polynomial_convert.vi"("Calib constants"=dbl[] [1.1471940648, -0.0162969407, 0.0008616246, -2.02143e-05, 1.764e-07], "Voltage"=w332) -> ("Eng Values"=w337:dbl)  [unwired: 4 in]
                    n157 = Equal To 0?(x=w332) -> (x = 0?=w331:bool)
                    n158 = In Range and Coerce(upper limit=1.12, x=w337, lower limit=0.88) -> (coerced(x)=w330:dbl)  [unwired: 1 out]
                    n159 = local read "Dem Road Speed"() -> (w327:dbl)
                    n160 = Select(t=0.88, s=w331, f=w330) -> (s? t:f=w329:dbl)
                    n161 = local read "Fan Control"() -> (w335:T2)
                    n162 = Bundle By Name(cluster=w335, "Set Wind Speed Ratio"=w329, "Set Fan Speed"=w327) -> (w334:T2)
                    n163 = local read "Fan Control REF"() -> (w333:refnum<k21>)
                    n164 = shared-variable-write(w333, w334) -> ()  [unwired: 1 in, 2 out]
                  }
                  frame #3 {
                    n165 = while {
                      shift-right: [w341] -> _
                      shift-left: _ -> [w342]
                      stop <- TRUE stop-if-true
                      n166 = local read "Working Section Temperature"() -> (w340:dbl)
                      n167 = Greater?(x=w340, y=35.0) -> (0:w341:bool)
                      n168 = Compound Arithmetic op=AND(invert w342, w341) -> (w347:bool)
                      n169 = Number To Fractional String(number=w340, precision (6)=i16 2) -> (F-format string=w344:string)  [unwired: 2 in]
                      n170 = case shown="True" w347 {
                        tunnel: w344 -> [_ w352]
                        frame False {
                        }
                        frame True {
                          w351 = string[] ["Aero_Tunnel:Fan:Watchdog", "Aero_Tunnel:Road:Watchdog", "Aero_Tunnel:Speed:Dem Velocity", "Aero_Tunnel:OGI Dem:Speed"] ("Channel Names")
                          n171 = Format Into String(format string="The Aero Tunnel temperature has gone above it's limits and is:\n%s\nThe Aero_Tunnel:Fan:Watchdog has therefore been disabled. ", w352) -> (resulting string=w353:string)  [unwired: 2 in, 1 out]
                          n172 = Bundle By Name(cluster=errorcluster {"status"=TRUE, "code"=0, "source"=""} ("error in (no error)"), "source"=w353) -> (w355:errorcluster)
                          n173 = Array Size(array=w351) -> (size(s)=w350:i32)
                          n174 = call "EnFlo_Error_Handler.vi"("error in (no error)"=w355, "Error Type"="Aero Tunnel Temperature Trip", "Dialog Box (T)"=FALSE) -> ()  [unwired: 3 out]
                          n175 = Initialize Array(0.0, w350) -> (w348:dbl[])
                          n176 = call "ASYNC_Adam_client.vi"("Values"=w348, "Channel Names"=w351) -> ()  [unwired: 2 out]
                        }
                      }
                    }
                  }
                }
              }
            }
          }
          frame #3 {
            # "10s Loop For Pulse"
            n177 = case shown="True" w360 {
              tunnel: w359 -> [_ w361]
              frame False {
                # "Do Nothing"
              }
              frame True {
                n178 = while {
                  shift-right: [w366] -> _
                  shift-left: "Start" -> [w367]
                  shift-right: [w365] -> _
                  shift-left: _ -> [w364]
                  tunnel: w361 -> [w363]
                  stop <- w368 continue-if-true
                  n179 = case shown="\"Close Server\"" w367 {
                    tunnel: [FALSE TRUE TRUE TRUE TRUE FALSE] -> w368
                    tunnel: ["" "Check Pulse" "Check Pulse" w408 "ReOpen" ""] -> w366
                    tunnel: [w369 w375 0 ("code") w400 w436 w445] -> w365
                    tunnel: w364 -> [w369 w376 _ w397 w436 w445]
                    tunnel: w363 -> [_ w379 _ _ _ _]
                    frame "No Match", Default {
                    }
                    frame "Start" {
                      n180 = Greater?(x=w379, y=1500) -> (0:w374:bool)
                      n181 = while {
                        shift-right: [w383] -> _
                        shift-left: _ -> [w382]
                        stop <- TRUE stop-if-true
                        n182 = Seconds To Date/Time() -> (date time rec=w384:T14)  [unwired: 2 in]
                        n183 = Unbundle By Name(w384) -> ("day of year"=w383:i32)
                        n184 = Not Equal?(x=w383, y=w382) -> (x != y?=w381:bool)
                        n185 = case shown="True" w381 {
                          frame False {
                          }
                          frame True {
                            n186 = Get Date/Time In Seconds() -> (seconds since 1Jan1904=w386:timestamp)
                            n187 = To Double Precision Float(number=w386) -> (double precision float=w385:dbl)
                            n188 = global write "Meas_global.vi" "Start Time of experiment"(w385) -> ()
                          }
                        }
                      }
                      n189 = Select(t=w376, s=w374, f=0) -> (s? t:f=w375:i32)
                    }
                    frame "ReOpen" {
                      n190 = local read "Paths"() -> (w393:path[])
                      n191 = call "Open_Remote_Vi.vi"("Run Minimised?"=bool[] [TRUE, FALSE], "Remote IP"="192.168.8.2", "Vi Path"=w393) -> ()  [unwired: 8 in, 1 out]
                      n192 = call "EnFlo_Error_Handler.vi"("error in (no error)"=errorcluster {"status"=TRUE, "code"=0, "source"="The Aero Server has just attempted to restart the OGI server on the ATE Machine "}, "Error Type"="ATE Machine Pulse Failure", "Dialog Box (T)"=FALSE) -> ()  [unwired: 3 out]
                    }
                    frame "Check Pulse" {
                      n193 = local read "ATE_Machine Status REF"() -> (w411:refnum<k21>)
                      n194 = shared-variable-read(w411) -> (w410:T5)  [unwired: 1 in, 3 out]
                      "ATE_Machine_Status" <- w410
                      n195 = Unbundle By Name(w410) -> ("Pulse"=w399:bool)
                      n196 = while {
                        shift-right: [w434] -> w401
                        shift-left: _ -> [w432]
                        tunnel: w399 -> [w434]
                        shift-left: _ -> [w433]
                        tunnel: [w433] -> w404
                        tunnel: [w432] -> w402
                        shift-left: _ -> [w431]
                        tunnel: [w431] -> w403
                        stop <- TRUE stop-if-true
                      }
                      n197 = Greater?(x=w397, y=3) -> (0:w398:bool)
                      n198 = Select(t=1.0, s=w399, f=0.0) -> (s? t:f=w413:dbl)
                      n199 = case shown="False" w398 {
                        tunnel: [FALSE w424] -> w405
                        tunnel: w404 -> [_ w423]
                        tunnel: w403 -> [_ w422]
                        tunnel: w402 -> [_ w421]
                        tunnel: w401 -> [_ w420]
                        frame False {
                        }
                        frame True {
                          n200 = Build Array(w420, w421, w423, w422) -> (w430:bool[])
                          n201 = Boolean Array To Number(Boolean array=w430) -> (number=w429:u32)
                          n202 = Equal?(x=u32 15, y=w429) -> (x = y?=w425:bool)
                          n203 = Equal?(x=w429, y=u32 0) -> (x = y?=w426:bool)
                          n204 = Or(x=w425, y=w426) -> (x .or. y?=w424:bool)
                        }
                      }
                      n205 = Bundle By Name(cluster=T9 {"Channel Name"="Aero_Tunnel:Server:Pulse", "New Value"=0.0} ("Update Scan Value Cluster"), "New Value"=w413) -> (w415:T9)
                      n206 = Build Array(w415) -> (w414:T9[])
                      n207 = call "Update_Current_Value_client.vi"("Don't Bother with check?"=TRUE, "Update array in"=w414) -> ()
                      n208 = Select(t="Close Server", s=w405, f="End") -> (s? t:f=w408:string)
                      n209 = Increment(x=w397) -> (x+1=w400:i32)
                    }
                    frame "Close Server" {
                      n210 = local read "Paths"() -> (w442:path[])
                      n211 = Index Array(array=w442) -> (element #1=w440:path, element #2=w439:path)  [unwired: 2 in]
                      n212 = call "Close_Remote_Vi.vi"("Also close host?"=FALSE, "Wait after host (ms)"=u32 2000, "Remote IP"="192.168.8.2", "Host Path"=w440, "VI Path"=w439) -> ()  [unwired: 6 in, 1 out]
                    }
                    frame "End" {
                    }
                  }
                }
              }
            }
          }
        }
        n213 = Or(x="Stop Button", y=w43) -> (x .or. y?=w41:bool)
        n214 = case shown="True" w45 {
          tunnel: w47 -> [w65 w90]
          tunnel: w59 -> [w68 w85]
          tunnel: w58 -> [_ w84]
          tunnel: [w66 i64 0 ("Period")] -> w44
          tunnel: w51 -> [w67 w76]
          tunnel: [w63 i64 1 ("Period")] -> w49
          tunnel: w48 -> [w64 w73]
          tunnel: [w68 i64 0 ("Global Start Time")] -> w46
          frame False {
            n215 = case shown="True" w65 {
              tunnel: w67 -> [w69 w71]
              tunnel: [w69 w70] -> w66
              frame False {
              }
              frame True {
                n216 = Increment(x=w71) -> (x+1=w70:i64)
              }
            }
            n217 = Increment(x=w64) -> (x+1=w63:i64)
          }
          frame True {
            n218 = Subtract(x=w85, y=w84) -> (x-y=w83:i64)
            n219 = To Double Precision Float(number=w76) -> (double precision float=w88:dbl)
            n220 = To Double Precision Float(number=w73) -> (double precision float=w78:dbl)
            n221 = To Double Precision Float(number=w83) -> (double precision float=w82:dbl)
            n222 = Divide(x=w88, y=w78) -> (x/y=w87:dbl)
            n223 = Multiply(x=w82, y=1e-09) -> (x*y=w80:dbl)
            n224 = Multiply(x=w87, y=100.0) -> (x*y=w74:dbl)
            n225 = Reciprocal(x=w80) -> (1/x=w79:dbl)
            n226 = Bundle By Name(cluster=T5 {"Loop Status"=FALSE, "Loop Frequency"=0.0, "Poor Loops"=0.0, "Pulse"=FALSE} ("ATE Machine Status"), "Loop Status"=w90, "Loop Frequency"=w79, "Poor Loops"=w74) -> (→"OGI Client Loop Status":T5)
          }
        }
        n227 = node-c288() -> ()  [unwired: 1 in, 1 out]
      }
      n228 = node-c288(w36) -> ()  [unwired: 1 out]
    }
    frame #3 {
      n229 = local read "ATE_Machine Status REF"() -> (w468:refnum<k21>)
      n230 = local read "Road Control REF"() -> (w463:refnum<k21>)
      n231 = local read "Balance Data REF"() -> (w467:refnum<k21>)
      n232 = local read "Fan Control REF"() -> (w466:refnum<k21>)
      n233 = local read "Road Data REF"() -> (w465:refnum<k21>)
      n234 = local read "Fan Data REF"() -> (w464:refnum<k21>)
      n235 = Close Variable Connection(11:w468) -> ()  [unwired: 1 in, 1 out]
      n236 = Close Variable Connection(11:w467) -> ()  [unwired: 1 in, 1 out]
      n237 = Close Variable Connection(11:w466) -> ()  [unwired: 1 in, 1 out]
      n238 = Close Variable Connection(11:w463) -> ()  [unwired: 1 in, 1 out]
      n239 = Close Variable Connection(11:w464) -> ()  [unwired: 1 in, 1 out]
      n240 = Close Variable Connection(11:w465) -> ()  [unwired: 1 in, 1 out]
      n241 = local read "Paths"() -> (w462:path[])
      n242 = Index Array(array=w462) -> (element #1=w460:path, element #2=w459:path)  [unwired: 2 in]
      n243 = call "Close_Remote_Vi.vi"("Also close host?"=TRUE, "Wait after host (ms)"=u32 2000, "Remote IP"="192.168.8.2", "Host Path"=w460, "VI Path"=w459) -> ()  [unwired: 6 in, 1 out]
    }
  }
